vi "RangeSearch.vi"() -> ()   [LabVIEW 2019]
panel:
  out "Input File":string
  in  "Input Path":path=path "C:/Users/jbrus/Documents/GitHub/LabVIEW/3LabVIEW-Specific-Features/RangeSearch/InputFileCSV.txt"
  in  "stop":bool
  out "RPM Output":dbl
  out "Array Index":dbl
  in  "Range":dbl(slide) scale=9.0..14.0
  out "Output Array":dbl[][](array[numeric])
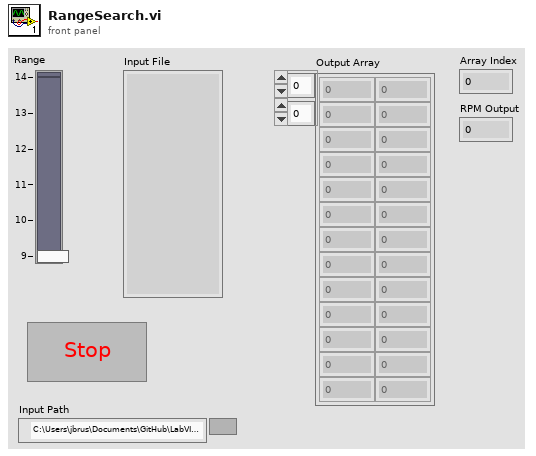
[diagram p1: front panel]
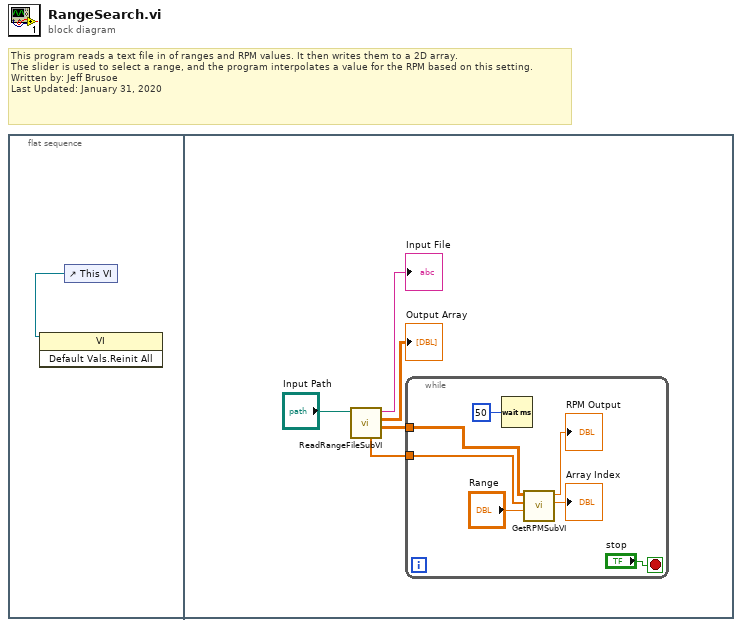
[diagram p0: block diagram]
diagram:
  # "This program reads a text file in of ranges and RPM values. It then writes them to a 2D array.\nThe slider is used to select a range, and the program interpolates a value for the RPM based on this setting.\nWritten by: Jeff Brusoe\nLast Updated: January 31, 2020"
  n1 = flat-sequence {
    frame #0 {
      n2 = control-ref of="This VI"() -> (w1:refnum<vi>)
      n3 = invoke class="VI" method="Default Vals.Reinit All"(reference=w1) -> ()  [unwired: 2 in, 3 out]
    }
    frame #1 {
      n4 = call "ReadRangeFileSubVI.vi"("Input Path"="Input Path") -> ("array type (2D Dbl) 2"=w6:dbl[][], "Output Array"=→"Output Array":dbl[][], "String"=→"Input File":string, "array type (2D Dbl)"=w5:dbl[])  [unwired: 6 in, 1 out]
      n5 = while {
        tunnel: w5 -> [w13]
        tunnel: w6 -> [w9]
        stop <- "stop" stop-if-true
        n6 = Wait (ms)(milliseconds to wait=u32 50) -> ()  [unwired: 1 out]
        n7 = call "GetRPMSubVI.vi"("Range"="Range", "array type (2D Dbl)"=w13, "array type (2D Dbl) 2"=w9) -> ("Array Index"=→"Array Index":dbl, "RPM Output"=→"RPM Output":dbl)  [unwired: 7 in]
      }
    }
  }
